vi "JSONRPC-GetCamerasInfo.vi"(11 "expId":string) -> (3 "Output":string[](array[string]))   [LabVIEW 2020]
uses:
  Configuration/Global_Configurations.vi
panel:
  # "GetCamerasInfo"
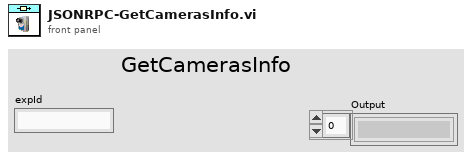
[diagram p1: front panel]
types:
  T1 = cluster{"Path":path, "Name":string, "Authors":string, "Keywords":string, "Description":string, "Cameras":cluster{"Base URL":string, "Path":string, "Name":string}[], "Sampling":cluster{"Sampled Variable":string, "Delta":dbl}[], "Sampling Freq":u32}[]
  T2 = cluster{"Base URL":string, "Path":string, "Name":string}[]
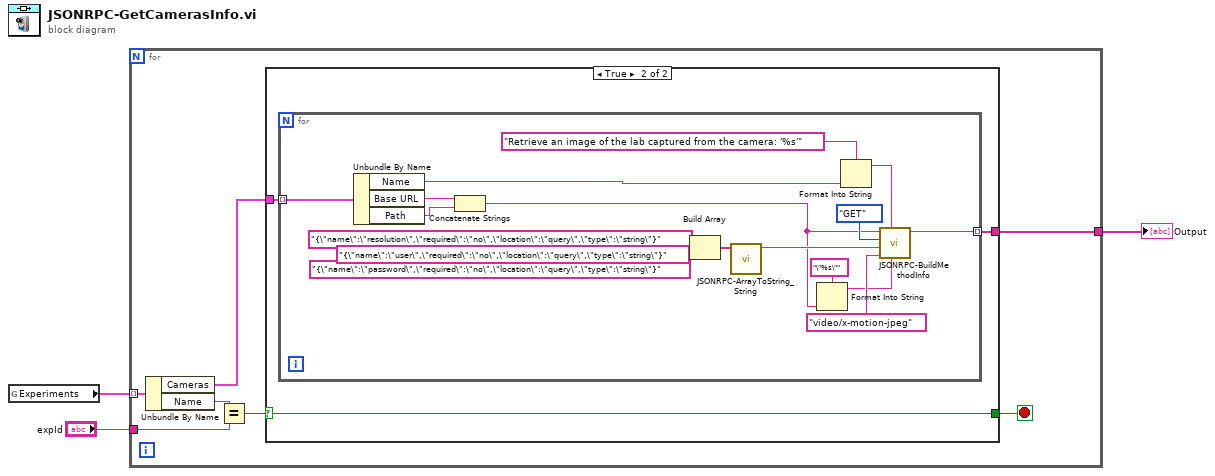
[diagram p0: block diagram]
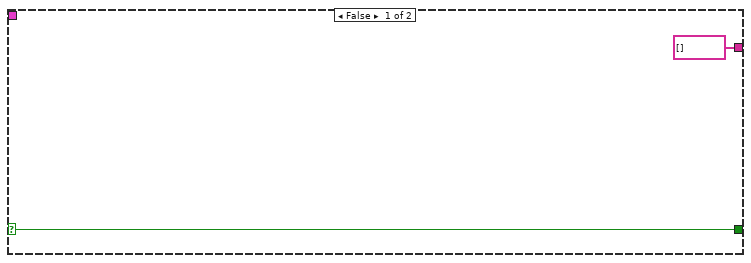
[diagram p2: hidden frame]
diagram:
  n1 = global read "Global_Configurations.vi" "Experiments"() -> (w3:T1)
  n2 = for {
    tunnel: w3 -> [w10] mode=indexing
    tunnel: "expId" -> [w8]
    tunnel: [w4] -> w1
    stop <- w6 stop-if-true
    n3 = Unbundle By Name(w10) -> ("Cameras"=w5:T2, "Name"=w9:string)
    n4 = Equal?(x=w9, y=w8) -> (x = y?=w7:bool)
    n5 = case shown="True" w7 {
      selector: w7 -> [w12 w15]
      tunnel: [w12 w15] -> w6
      tunnel: w5 -> [_ w14]
      tunnel: [string[] [] w13] -> w4
      frame False {
      }
      frame True {
        n6 = for {
          tunnel: [w26] -> w13 mode=indexing
          tunnel: w14 -> [w19] mode=indexing
          n7 = Unbundle By Name(w19) -> ("Name"=w16:string, "Base URL"=w18:string, "Path"=w17:string)
          n8 = Concatenate Strings(w18, w17) -> (w20:string)
          n9 = Build Array("{\"name\":\"resolution\",\"required\":\"no\",\"location\":\"query\",\"type\":\"string\"}" ("Params"), "{\"name\":\"user\",\"required\":\"no\",\"location\":\"query\",\"type\":\"string\"}" ("Params"), "{\"name\":\"password\",\"required\":\"no\",\"location\":\"query\",\"type\":\"string\"}" ("Params")) -> (w28:string[])
          n10 = call "JSONRPC-ArrayToString_String.vi"("Array"=w28) -> ("Output"=w23:string)  [unwired: 10 in]
          n11 = Format Into String(format string="\"%s\"", w20) -> (resulting string=w22:string)  [unwired: 2 in, 1 out]
          n12 = Format Into String(format string="Retrieve an image of the lab captured from the camera: '%s'" ("Description"), w16) -> (resulting string=w21:string)  [unwired: 2 in, 1 out]
          n13 = call "JSONRPC-BuildMethodInfo.vi"("Example"=w22, "Description"=w21, "Returns"="video/x-motion-jpeg", "Params"=w23, "Method"=enum16{"SSE", "GET", "POST"}."GET", "url"=w20) -> ("String"=w26:string)  [unwired: 5 in]
        }
      }
    }
  }
  "Output" <- w1
